vi "Demo2.vi"() -> ()   [LabVIEW 2016]
uses:
  IPopulation/IPopulation.lvclass
  Numeric Optimization/Gene/Bit.lvclass
  C:/Users/J51654/My Projects/Evolutionary Programming/GA Framework/IGene/IGene.lvclass
  Numeric Optimization/Chromosome/Solution.lvclass
  C:/Users/J51654/My Projects/Evolutionary Programming/GA Framework/IChromosome/IChromosome.lvclass
  IPopulation/IPopulation.lvclass/IPopulation.ctl
  IChromosome/IChromosome.lvclass/IChromosome.ctl
  Numeric Optimization/Gene/Bit.lvclass/Bit.ctl
  IChromosome/IChromosome.lvclass
  IGene/IGene.lvclass
panel:
  out "Average Fitness":dbl
  out "Waveform Graph":dbl[](graph)
  out "Best Fit":dbl
  out "Generations":i32
  # "TARGET SOLUTION = 5.0"
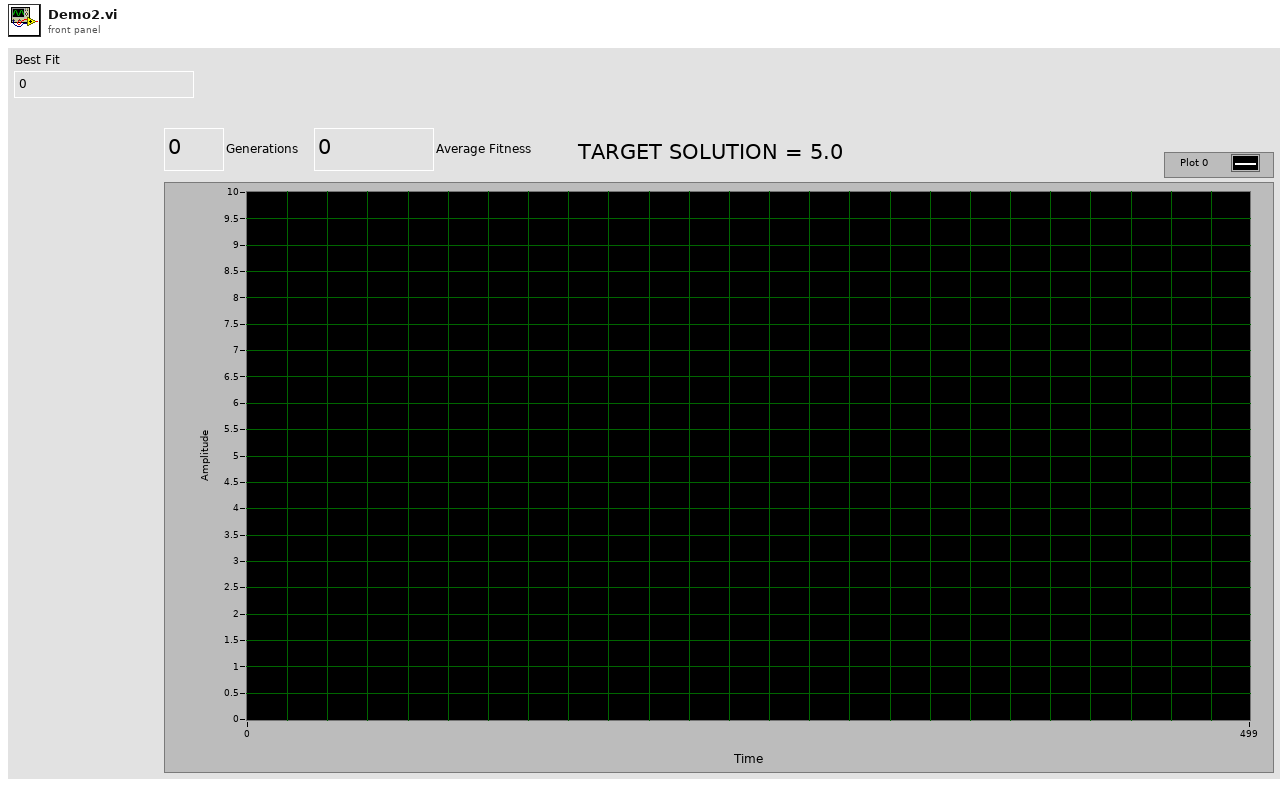
[diagram p1: front panel]
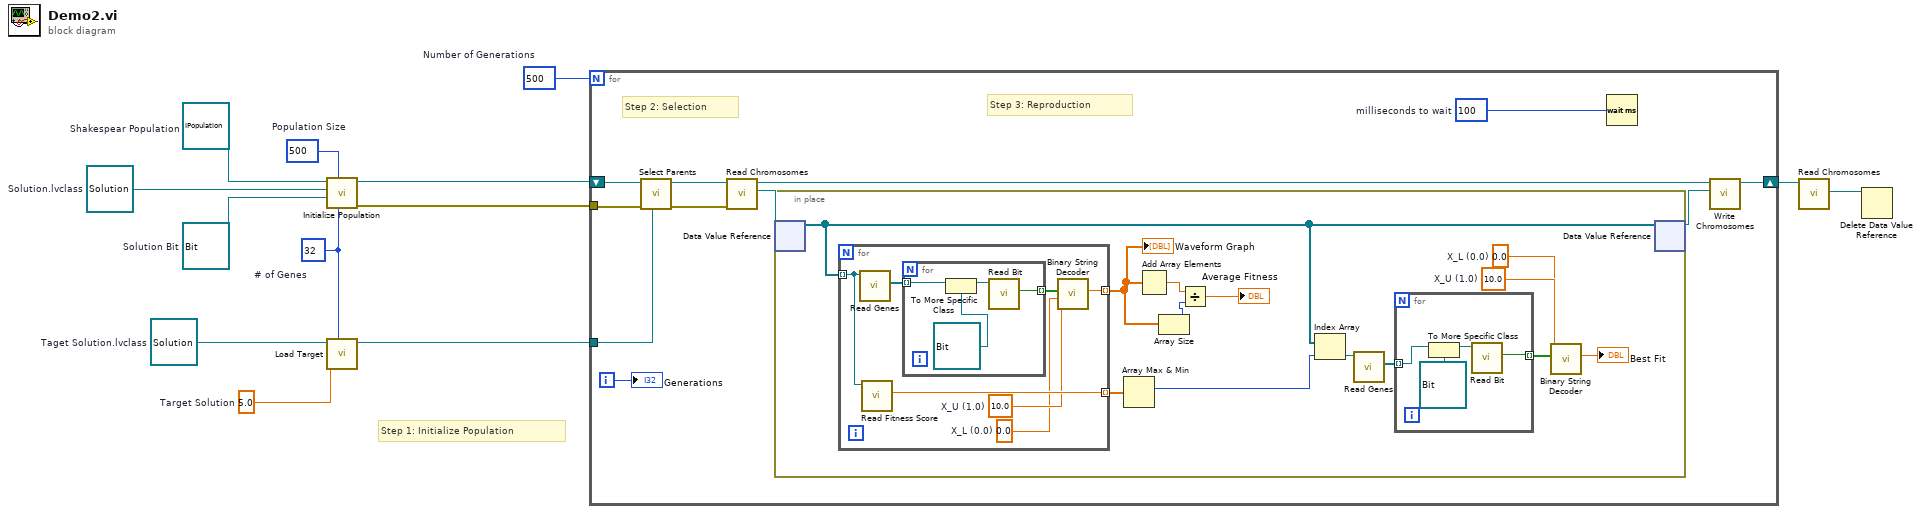
[diagram p0: block diagram]
diagram:
  w2 = refnum<class "Solution.lvclass"> refnum  # Solution.lvclass
  w3 = 5.0  # Target Solution
  w4 = u32 32  # # of Genes
  w6 = refnum<class "Solution.lvclass"> refnum  # Taget Solution.lvclass
  w7 = refnum<class "Bit.lvclass"> refnum  # Solution Bit
  w10 = 500  # Number of Generations
  w12 = u32 500  # Population Size
  w13 = refnum<class "IPopulation.lvclass"> refnum  # Shakespear Population
  # "Step 1: Initialize Population"
  n1 = call "Initialize Population.vi"("# of Genes"=w4, "Population Size"=w12, "Gene Type"=w7, "Chromosome Type"=w2, "IPopulation in"=w13) -> ("error out"=w11:errorcluster, "IPopulation out"=w1:refnum<class "IPopulation.lvclass">)  [unwired: 5 in]
  n2 = call "Load Target.vi"("Number of Bits (n)"=w4, "Target String"=w3, "Sentence in"=w6) -> ("Sentence out"=w5:refnum<class "Solution.lvclass">)  [unwired: 7 in, 1 out]
  n3 = for {
    N: w10 -> [_]
    tunnel: w5 -> [w15]
    tunnel: w11 -> [w23]
    shift-right: [w18] -> w9
    shift-left: w1 -> [w24]
    i -> [w22]
    w14 = u32 100  # milliseconds to wait
    # "Step 3: Reproduction"
    # "Step 2: Selection"
    n4 = call "Select Parents.vi"("Target Chromosome"=w15, "error in"=w23, "IPopulation in"=w24) -> ("error out"=w16:errorcluster, "IPopulation out"=w21:refnum<class "IPopulation.lvclass">)  [unwired: 7 in]
    n5 = call "Read Chromosomes.vi"("error in (no error)"=w16, "IPopulation in"=w21) -> ("Chromosomes"=w20:refnum<data-value>, "IPopulation out"=w19:refnum<class "IPopulation.lvclass">)  [unwired: 7 in, 1 out]
    n6 = in-place {
      w29 = 0.0  # X_L (0.0)
      w30 = 10.0  # X_U (1.0)
      n7 = in-place-dvr #1(w20) -> (w36:refnum<class "IChromosome.lvclass">[])  [unwired: 1 out]
      n8 = for {
        tunnel: w36 -> [w47] mode=indexing
        tunnel: [w44] -> w28 mode=indexing
        tunnel: [w46] -> w37 mode=indexing
        w42 = 0.0  # X_L (0.0)
        w43 = 10.0  # X_U (1.0)
        n9 = call "Read Genes.vi"("IChromosome in"=w47) -> ("Genes"=w48:refnum<class "IGene.lvclass">[])  [unwired: 8 in, 2 out]
        n10 = call "Read Fitness Score.vi"("IChromosome in"=w47) -> ("Fitness Score"=w46:dbl)  [unwired: 8 in, 2 out]
        n11 = for {
          tunnel: w48 -> [w52] mode=indexing
          tunnel: [w49] -> w45 mode=indexing
          n12 = To More Specific Class(target class=refnum<class "Bit.lvclass"> refnum ("Bit.lvclass"), reference=w52) -> (specific class reference=w50:refnum<class "Bit.lvclass">)  [unwired: 1 in, 1 out]
          n13 = call "Read Bit.vi"("Bit in"=w50) -> ("Bit"=w49:bool)  [unwired: 8 in, 2 out]
        }
        n14 = call "Binary String Decoder.vi"("X_L (0.0)"=w42, "Binary String (LSb[0] - MSb[n-1])"=w45, "X_U (1.0)"=w43) -> ("x"=w44:dbl)  [unwired: 8 in]
      }
      "Waveform Graph" <- w28
      n15 = Array Max & Min(array=w37) -> (max index (indices)=w35:i32)  [unwired: 3 out]
      n16 = Add Array Elements(numeric array=w28) -> (sum=w26:dbl)
      n17 = Array Size(array=w28) -> (size(s)=w27:i32)
      n18 = Divide(x=w26, y=w27) -> (x/y=→"Average Fitness":dbl)
      n19 = Index Array(array=w36, index=w35) -> (element=w34:refnum<class "IChromosome.lvclass">)
      n20 = call "Read Genes.vi"("IChromosome in"=w34) -> ("Genes"=w33:refnum<class "IGene.lvclass">[])  [unwired: 8 in, 2 out]
      n21 = for {
        tunnel: w33 -> [w39] mode=indexing
        tunnel: [w38] -> w32 mode=indexing
        n22 = To More Specific Class(target class=refnum<class "Bit.lvclass"> refnum ("Bit.lvclass"), reference=w39) -> (specific class reference=w40:refnum<class "Bit.lvclass">)  [unwired: 1 in, 1 out]
        n23 = call "Read Bit.vi"("Bit in"=w40) -> ("Bit"=w38:bool)  [unwired: 8 in, 2 out]
      }
      n24 = call "Binary String Decoder.vi"("X_L (0.0)"=w29, "Binary String (LSb[0] - MSb[n-1])"=w32, "X_U (1.0)"=w30) -> ("x"=→"Best Fit":dbl)  [unwired: 8 in]
      n25 = in-place-dvr #1(w36) -> (w17:refnum<data-value>)  [unwired: 1 out]
    }
    n26 = Wait (ms)(milliseconds to wait=w14) -> ()  [unwired: 1 out]
    n27 = call "Write Chromosomes.vi"("Chromosomes"=w17, "IPopulation in"=w19) -> ("IPopulation out"=w18:refnum<class "IPopulation.lvclass">)  [unwired: 8 in, 1 out]
    "Generations" <- w22
  }
  n28 = call "Read Chromosomes.vi"("IPopulation in"=w9) -> ("Chromosomes"=w8:refnum<data-value>)  [unwired: 8 in, 2 out]
  n29 = Delete Data Value Reference(data value reference=w8) -> ()  [unwired: 1 in, 2 out]
